vi "startTestSeries.vi"(0 "EnabledState in":refnum<class "WaitingForTestState.lvclass">, 1 "Model in":refnum<class "Model.lvclass">, 2 "Serial Number":string, 3 "Operator":string, 4 "Comments":string, 5 "error in (no error)":errorcluster) -> (14 "EnabledState out":refnum<class "WaitingForTestState.lvclass">, 15 "Model out":refnum<class "Model.lvclass">, 19 "error out":errorcluster)   [LabVIEW 2015, in "WaitingForTestState.lvclass"]
uses:
  WaitingForTestState.lvclass
  Model/Model/Model.lvclass
  Typedefs/StateSelector.ctl
  Typedefs/ILCBTTypedefs.lvlib
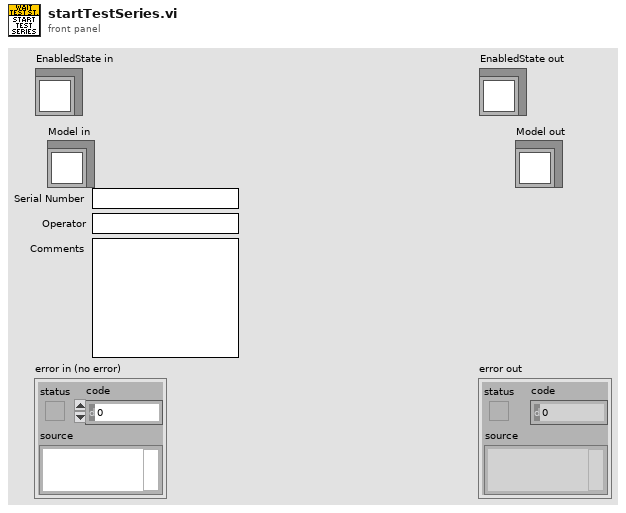
[diagram p1: front panel]
types:
  T1 = typedef "ILCBTTypedefs.lvlib/StateSelector.ctl" = enum16{"EnabledState", "FaultState", "OffState", "StandbyState", "WaitingForTestState", "ExecutingTestState"}
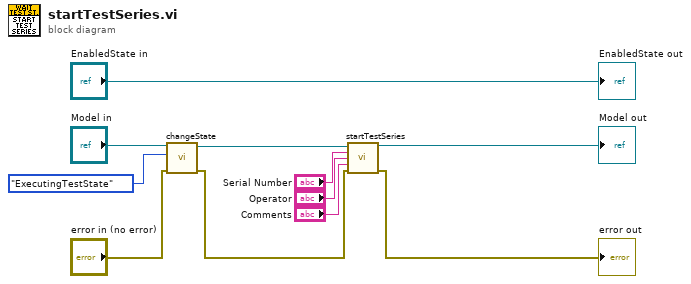
[diagram p0: block diagram]
diagram:
  n1 = call "changeState.vi"("error in (no error)"="error in (no error)", "State:"=StateSelector."ExecutingTestState", "Model in"="Model in") -> ("error out"=w2:errorcluster, "Model out"=w4:refnum<class "Model.lvclass">)  [unwired: 7 in]
  n2 = call "startTestSeries.vi"("Model in"=w4, "Serial Number"="Serial Number", "Operator"="Operator", "Comments"="Comments", "error in (no error)"=w2) -> ("Model out"=→"Model out":refnum<class "Model.lvclass">, "error out"=→"error out":errorcluster)  [unwired: 9 in]
  "EnabledState out" <- "EnabledState in"
